vi "Wait for reachability.vi"(7 "timeout (ms)":i32, 8 "error in (no error)":errorcluster, 10 "must be directly reachable?":bool, 11 "address":refnum<class "mDNS Hostname Network Address.lvclass">) -> (0 "error out":errorcluster, 2 "found?":bool, 3 "address out":refnum<class "Generic Network Address.lvclass">)   [LabVIEW 2020, in "NI_WFCN.lvlib" / "mDNS Hostname Network Address.lvclass"]
doc: "mDNS is assumed to always be configured, so this redirects into Test for reachability.vi, which will always succeed."
uses:
  <vilib>/net/WFCN/Addressing/mDNS Hostname Network Address/mDNS Hostname Network Address.lvclass
  <vilib>/net/WFCN/Addressing/Generic Network Address/Generic Network Address.lvclass
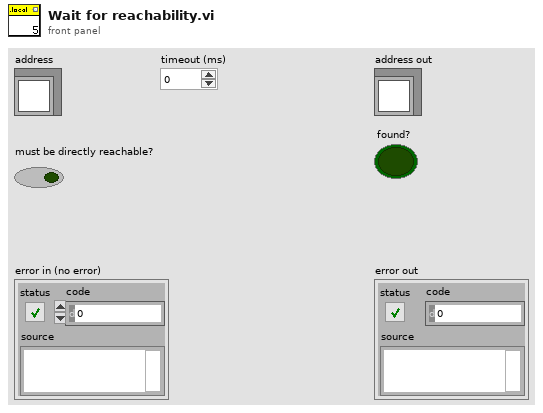
[diagram p1: front panel]
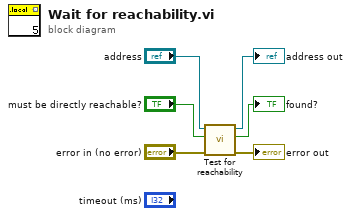
[diagram p0: block diagram]
diagram:
  n1 = call-dynamic "Test for reachability.vi"("error in (no error)"="error in (no error)", "must be directly reachable?"="must be directly reachable?", "address"="address") -> ("error out"=→"error out":errorcluster, "found?"=→"found?":bool, "address out"=→"address out":refnum<class "Generic Network Address.lvclass">)  [unwired: 6 in]
